vi "Name to User Event.vi"(0 "User Event Name":string) -> (1 "Is Registered?":bool, 5 "Found?":bool, 6 "User Event":refnum<user-event>)   [LabVIEW 2021, in "UserEvent.lvlib"]
uses:
  UserEvent.lvlib
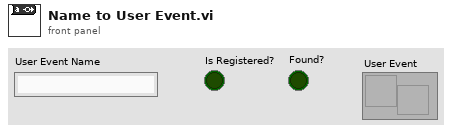
[diagram p1: front panel]
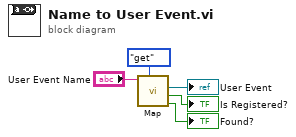
[diagram p0: block diagram]
diagram:
  n1 = call "Map.vi"("Action"=enum8{"noop", "get", "set", "pop"}."get", "User Event Name"="User Event Name") -> ("Found?"=→"Found?":bool, "Is Registered out"=→"Is Registered?":bool, "User Event out"=→"User Event":refnum<user-event>)  [unwired: 6 in, 1 out]
